vi "Read Dictionary Element.vi"(8 "error in (no error)":errorcluster, 10 "key":string, 11 "Control Experiment in":refnum<class "Control Experiment.lvclass">) -> (0 "error out":errorcluster, 2 "value":variant, 3 "Control Experiment out":refnum<class "Control Experiment.lvclass">)   [LabVIEW 2019, in "Control Experiment.lvclass"]
uses:
  Control Experiment.lvclass
  Control Experiment.lvclass/Control Experiment.ctl
  <userlib>/LevyLab/LV-Data/LV-Data/LV-Data.lvclass
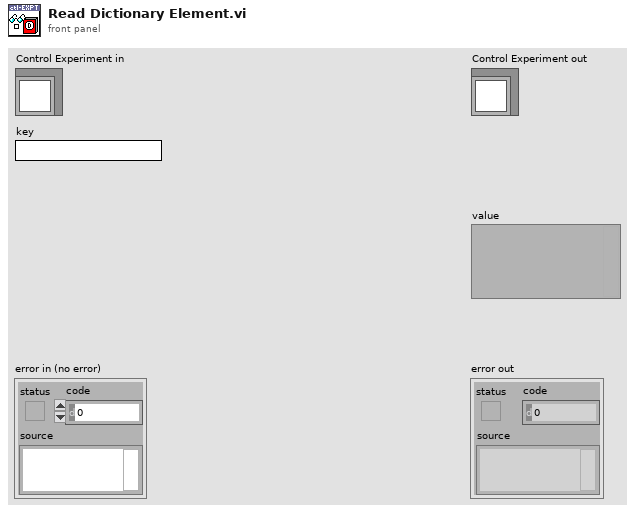
[diagram p1: front panel]
types:
  T1 = typedef "Dictionary Object RefNum__ogtk.ctl" = refnum<k1>
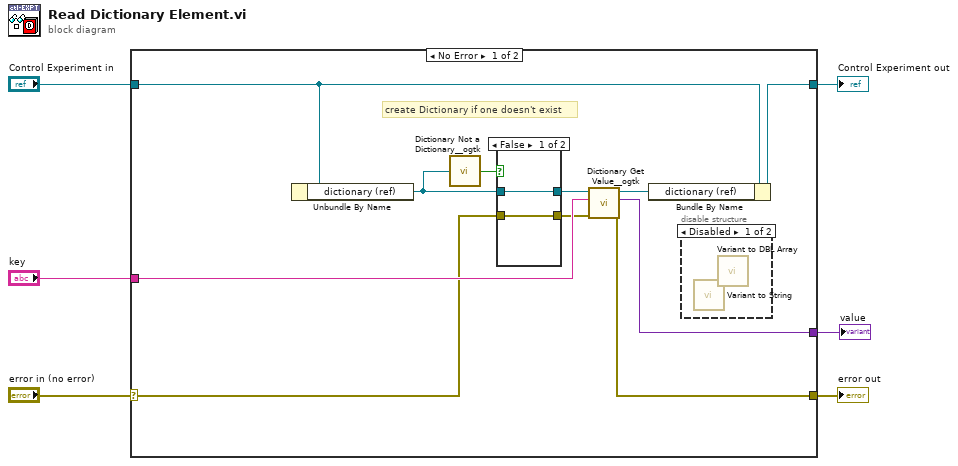
[diagram p0: block diagram]
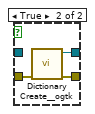
[diagram p3: hidden frame]
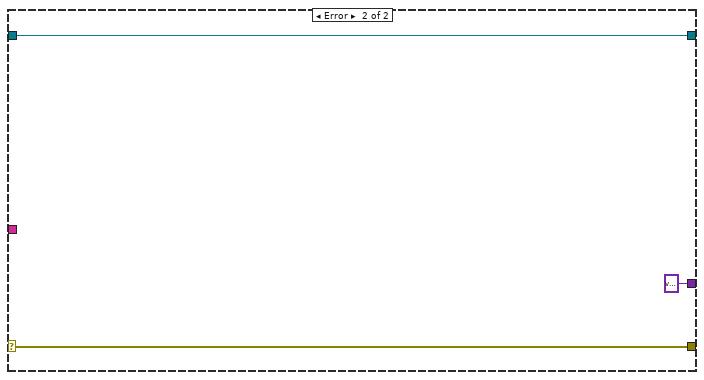
[diagram p4: hidden frame]
diagram:
  n1 = case shown="No Error" "error in (no error)" {
    selector: "error in (no error)" -> [w9 w24]
    tunnel: [w7 w24] -> w5
    tunnel: [w17 w25] -> w3
    tunnel: "Control Experiment in" -> [w16 w25]
    tunnel: "key" -> [w11 _]
    tunnel: [w8 variant ("value")] -> w1
    frame No Error {
      # "create Dictionary if one doesn't exist"
      n2 = Unbundle By Name(w16) -> ("dictionary (ref)"=w14:T1)
      n3 = call <userlib>:"Dictionary Not a Dictionary__ogtk.vi"("dictionary"=w14) -> ("not a dictionary?"=w15:bool)
      n4 = case shown="False" w15 {
        tunnel: [w19 w22] -> w13
        tunnel: w14 -> [w19 _]
        tunnel: [w18 w21] -> w10
        tunnel: w9 -> [w18 w20]
        frame False {
        }
        frame True {
          n5 = call <userlib>:"Dictionary Create__ogtk.vi"("error in (no error)"=w20) -> ("error out"=w21:errorcluster, "dictionary out"=w22:T1)  [unwired: 9 in]
        }
      }
      n6 = call <userlib>:"Dictionary Get Value__ogtk.vi"("error in"=w10, "key"=w11, "dictionary"=w13) -> ("error out"=w7:errorcluster, "value"=w8:variant, "dictionary out"=w12:T1)  [unwired: 5 in, 1 out]
      n7 = Bundle By Name(cluster=w16, "dictionary (ref)"=w12) -> (w17:refnum<class "Control Experiment.lvclass">)
      n8 = disable-structure shown="Disabled" {
        frame Disabled {
          n9 = call <userlib>:"Variant to String.vi"() -> ()  [unwired: 10 in, 2 out]
          n10 = call "Variant to DBL Array.vi"() -> ()  [unwired: 10 in, 2 out]
        }
        frame Enabled {
        }
      }
    }
    frame Error {
    }
  }
  "error out" <- w5
  "Control Experiment out" <- w3
  "value" <- w1
